vi "Begin.vi"(8 "error in":errorcluster) -> (0 "error out":errorcluster)   [LabVIEW 2019]
doc: "Called before other user functions, this VI is expected to open initial I/O refnums, load in file data, and do all program initialization. Notice that the <B>error out</B> terminal is simply used for data flow. Wiring it to other structures or subVIs ensures that this VI runs first."
uses:
  <vilib>/Rock Robotics/WPI/Camera/WPI_CameraImageSize.ctl
  <vilib>/Rock Robotics/WPI/DriverStation/WPI_DriverStationRobotMode2.ctl
  <vilib>/Rock Robotics/WPI/Joystick/WPI_JoystickDeviceEnum.ctl
  <vilib>/Rock Robotics/SystemInterfaces/DIO/FPGA_DIOChannel.ctl
  <vilib>/Rock Robotics/WPI/Encoder/WPI_EncoderType.ctl
  <vilib>/Rock Robotics/WPI/Solenoid/WPI_SolenoidChannel.ctl
  <vilib>/Rock Robotics/WPI/Solenoid/WPI_SolenoidValue.ctl
  <vilib>/Rock Robotics/WPI/SafetyOutput/WPI_SafetyOutputConfigMenu.ctl
  <vilib>/Rock Robotics/WPI/Camera/WPI_CameraFrameRate.ctl
  <vilib>/Rock Robotics/WPI/Camera/WPI_CameraWhite Balance Values.ctl
  <vilib>/Rock Robotics/WPI/Camera/WPI_CameraExposure Values.ctl
  Robot Global Data.vi
  <vilib>/Rock Robotics/Network Tables/NT Write String Array.vi
  <vilib>/Rock Robotics/WPI/Counter/WPI_CounterDigitalInputToDigitalSource.vi
  <vilib>/Rock Robotics/WPI/Solenoid/WPI_SolenoidOpenDouble.vi
  <vilib>/Rock Robotics/WPI/Solenoid/WPI_SolenoidSetEnum.vi
  <vilib>/Rock Robotics/WPI/RobotDrive/WPI_RobotDriveOpen4MotorWithExistingMotors.vi
  <vilib>/Rock Robotics/WPI/Utilities/WPI_GetSetVariantRefNum.vi
panel:
  in  "Image Size":T1=enum."320x240"
  in  "Image Size 2":T1=enum."320x240"
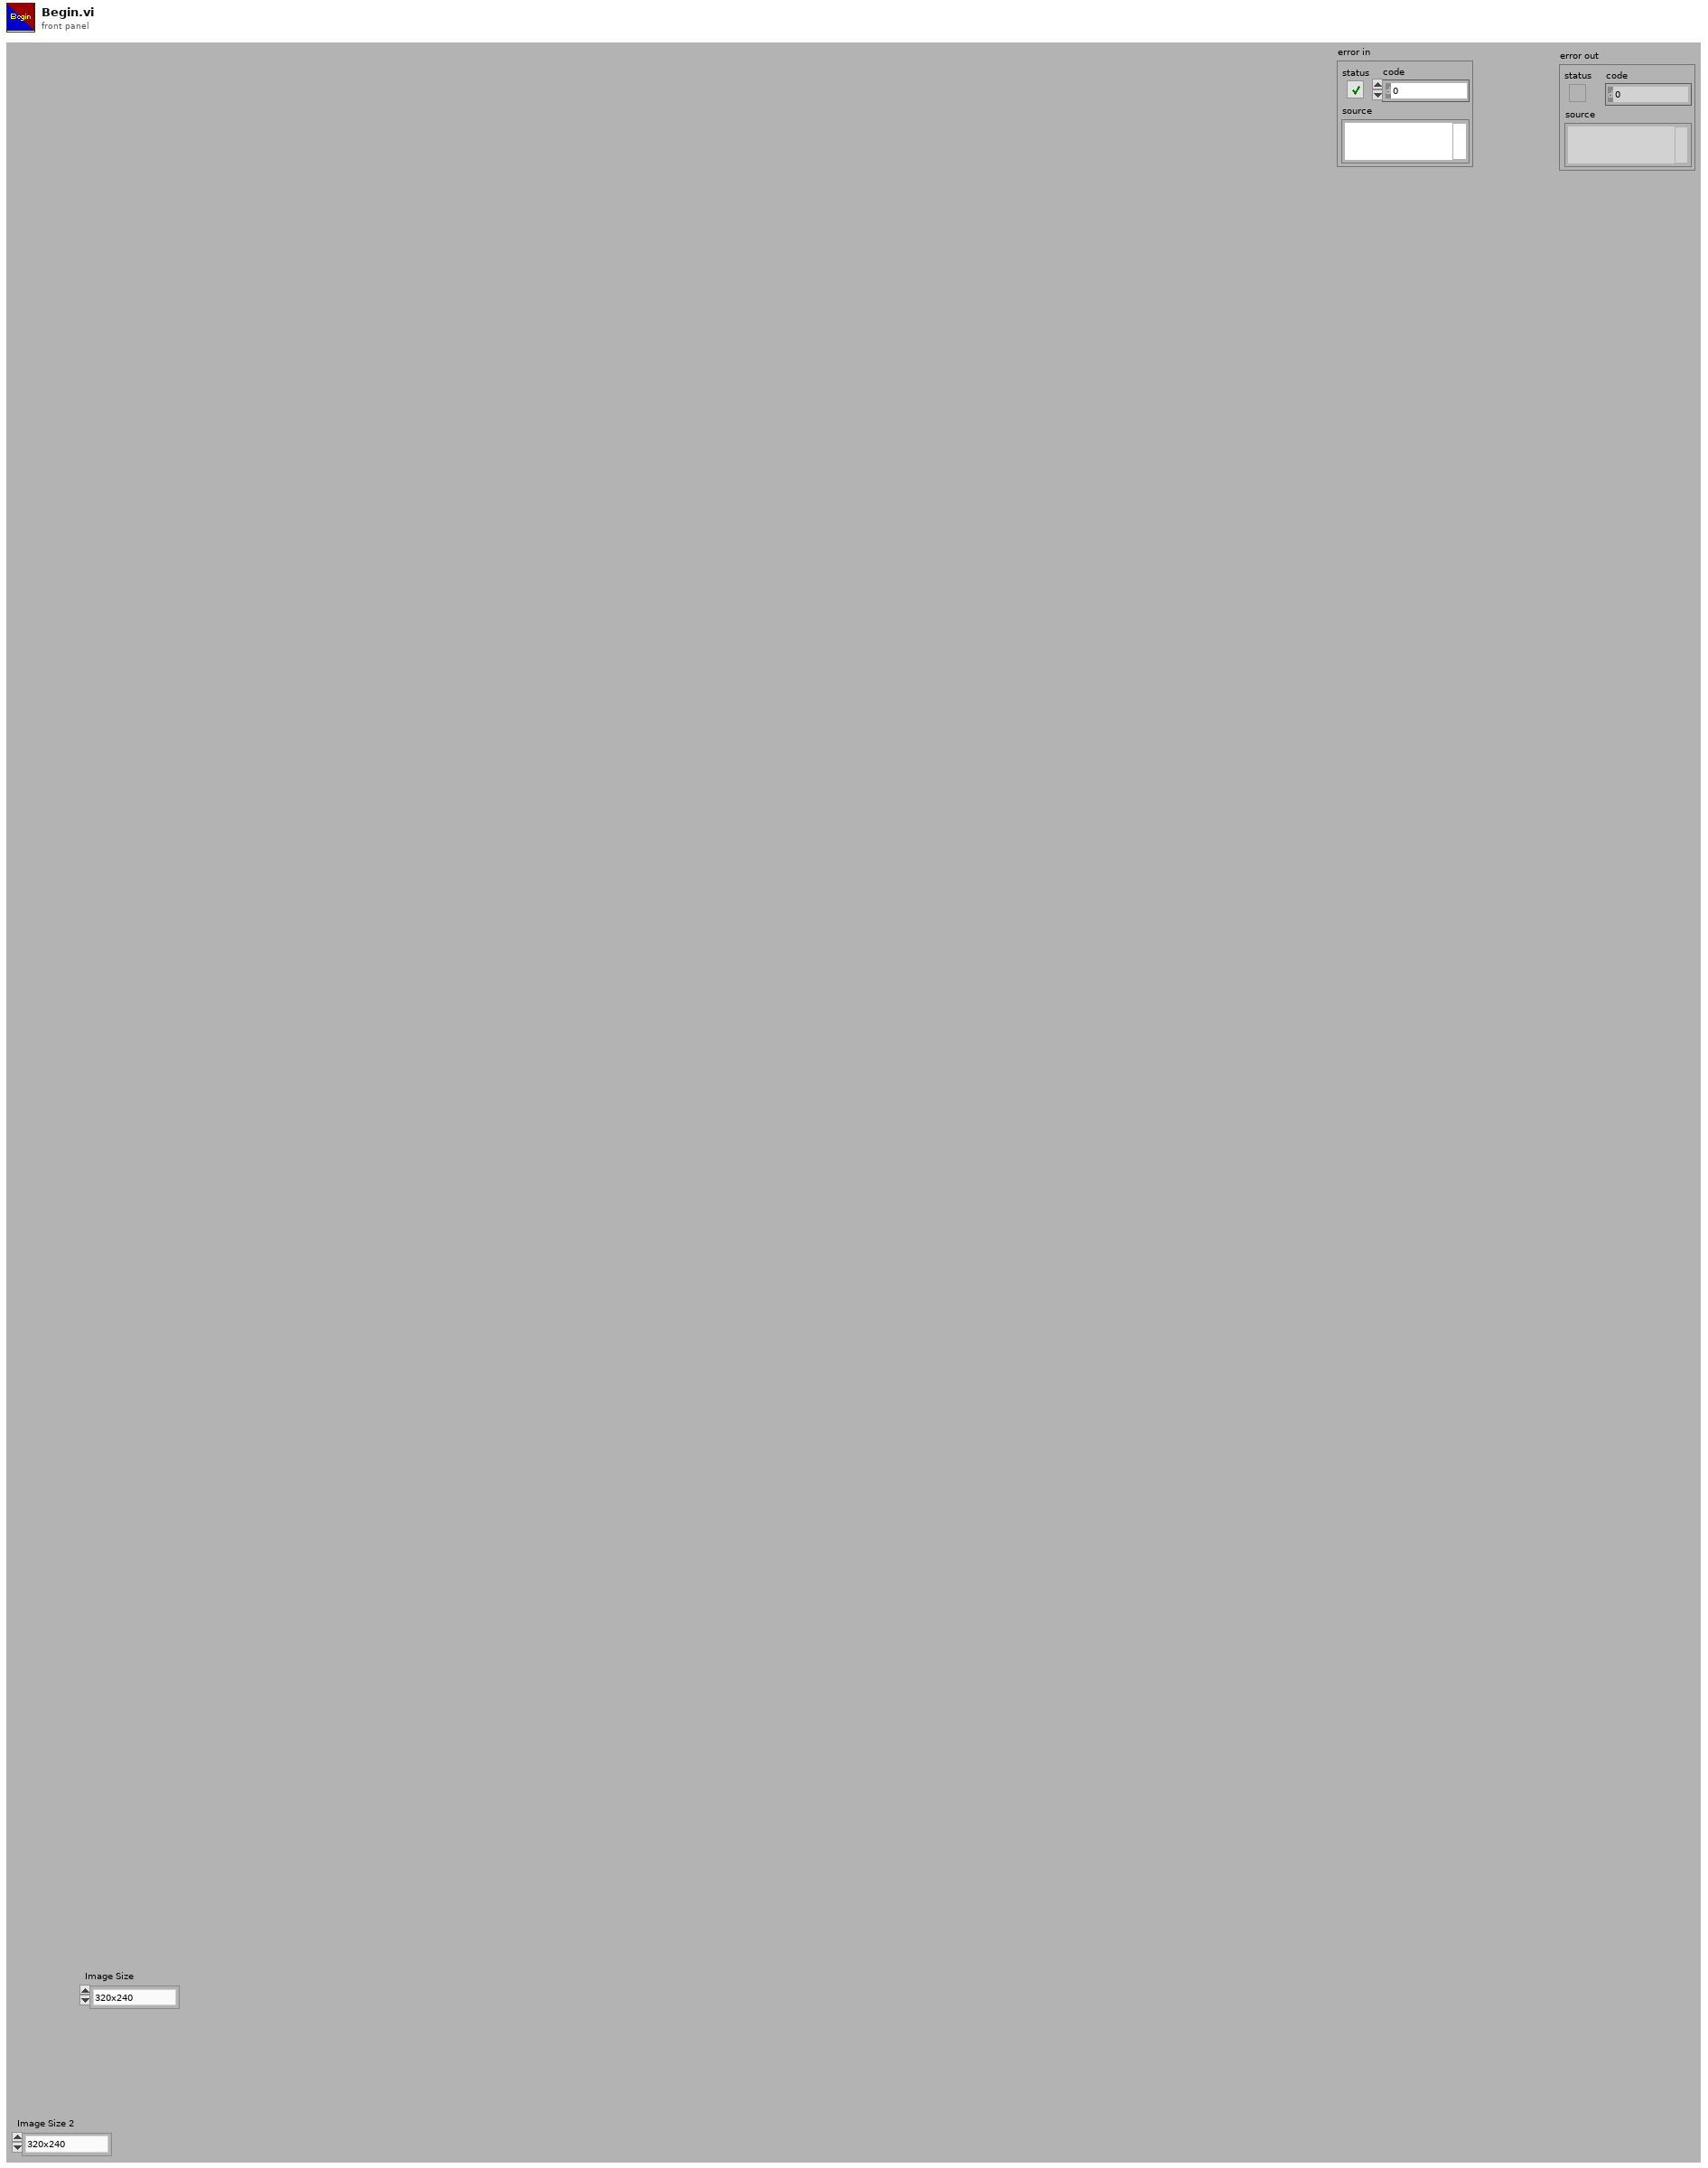
[diagram p1: front panel]
types:
  T1 = typedef "WPI_CameraImageSize.ctl" = enum16{"640x480", "320x240", "160x120", "Custom"}
  T2 = typedef "WPI_CameraFrameRate.ctl" = u32
  T3 = typedef "WPI_CameraExposure Values.ctl" = enum16{"Auto", "Flicker-free 50 Hz", "Flicker-free 60 Hz", "Hold current", "Custom"}
  T4 = typedef "WPI_CameraWhite Balance Values.ctl" = enum16{"Auto", "Fixed indoor", "Fixed outdoor 1", "Fixed outdoor 2", "Fixed fluorescent 1", "Fixed fluorescent 2", "Hold current", "Custom"}
  T5 = typedef "WPI_SolenoidValue.ctl" = enum16{"Off", "On", "Forward", "Reverse"}
  T6 = typedef "WPI_SolenoidChannel.ctl" = enum8{"Solenoid 0", "Solenoid 1", "Solenoid 2", "Solenoid 3", "Solenoid 4", "Solenoid 5", "Solenoid 6", "Solenoid 7", "Invalid"}
  T7 = typedef "WPI_JoystickDeviceEnum.ctl" = enum16{"USB 0", "USB 1", "USB 2", "USB 3", "USB 4", "USB 5"}
  T8 = typedef "WPI_SafetyOutputConfigMenu.ctl" = enum16{"Enable", "Disable"}
  T9 = typedef "WPI_EncoderType.ctl" = enum16{"1x", "2x", "4x"}
  T10 = typedef "FPGA_DIOChannel.ctl" = enum8{"DIO 0", "DIO 1", "DIO 2", "DIO 3", "DIO 4", "DIO 5", "DIO 6", "DIO 7", "DIO 8", "DIO 9", "DIO MXP 0", "DIO MXP 1", "DIO MXP 2", "DIO MXP 3", "DIO MXP 4", "DIO MXP 5", "DIO MXP 6", "DIO MXP 7", "DIO MXP 8", "DIO MXP 9", "DIO MXP 10", "DIO MXP 11", "DIO MXP 12", "DIO MXP 13", "DIO MXP 14", "DIO MXP 15", "SPI Port CS1", "SPI Port CS2", "SPI Port CS3", "SPI Port MISO", "SPI Port MOSI", "Invalid"}
  T11 = typedef "WPI_DriverStationRobotMode2.ctl" = enum16{"Autonomous Disabled", "Autonomous Enabled", "Teleop Disabled", "Teleop Enabled", "Disconnected", "Finish", "Test Disabled", "Test Enabled", "Emergency Stopped"}
  T12 = typedef "WPI_JoystickDevRef.ctl" = cluster{"Device":T7}
  T13 = typedef "WPI_SolenoidDevRef.ctl" = cluster{"DevStatus":errorcluster, "Pneumatics Control Module":u8, "Forward Solenoid Channel":T6, "Reverse Solenoid Channel":T6}
  T14 = typedef "WPI_CameraDevRef.ctl" = cluster{"Camera Address":string, "CameraStatus":errorcluster}
  T15 = typedef "WPI_MotorControlDeviceRef.ctl" = cluster{"DeviceStatus":errorcluster, "Type":T16, "PWM":cluster{"PWM Channel":T17, "DeadBand":T18}, "CAN":cluster{"Device Number":u8, "SetOutput VI Ref":variant, "GetOutput VI Ref":variant, "Enable VI Ref":variant, "Disable VI Ref":variant, "Data":variant}, "Invert":bool, "DIO PWM":cluster{"PWM \"Enable\" Channel":T17, "DIOChannel":T10, "PWM Rate":dbl}}
  T16 = typedef "WPI_MotorControlType.ctl" = enum16{"PWM", "CAN", "DIO PWM"}
  T17 = typedef "FPGA_DIOPWMChannel.ctl" = enum8{"PWM 0", "PWM 1", "PWM 2", "PWM 3", "PWM 4", "PWM 5", "PWM 6", "PWM 7", "PWM 8", "PWM 9", "PWM MXP 0", "PWM MXP 1", "PWM MXP 2", "PWM MXP 3", "PWM MXP 4", "PWM MXP 5", "PWM MXP 6", "PWM MXP 7", "PWM MXP 8", "PWM MXP 9", "Invalid"}
  T18 = typedef "WPI_PWMDeadband.ctl" = cluster{"Name":string, "maxPositivePwm":i32, "minPositivePwm":i32, "centerPwm":i32, "maxNegativePwm":i32, "minNegativePwm":i32, "angularRange":u16}
  T19 = typedef "WPI_CompressorDevRef.ctl" = cluster{"DevStatus":errorcluster, "Pneumatics Control Module":u8}
  T20 = typedef "WPI_DigitalInputDevRef.ctl" = cluster{"DevStatus":errorcluster, "DIO Channel":T10}
  T21 = typedef "WPI_RobotDriveDevRef.ctl" = cluster{"DevStatus":errorcluster, "Motors[]":T15[], "Square Inputs":bool, "Max Output":dbl}
  T22 = typedef "FPGA_CounterEncoderSourceConvertionLVSourceType.ctl" = cluster{"DevStatus":errorcluster, "AnalogTriggerMode?":bool, "DigitalMode":cluster{"DIO Channel":T23}, "AnalogTriggerMode":cluster{"AnalogTriggerIndex":T24, "OutputType":T25}}
  T23 = typedef "FPGA_DIODigitalSourceChannel.ctl" = enum8{"DIO 0", "DIO 1", "DIO 2", "DIO 3", "DIO 4", "DIO 5", "DIO 6", "DIO 7", "DIO 8", "DIO 9", "DIO MXP 0", "DIO MXP 1", "DIO MXP 2", "DIO MXP 3", "DIO MXP 4", "DIO MXP 5", "DIO MXP 6", "DIO MXP 7", "DIO MXP 8", "DIO MXP 9", "DIO MXP 10", "DIO MXP 11", "DIO MXP 12", "DIO MXP 13", "DIO MXP 14", "DIO MXP 15", "SPI Port CS1", "SPI Port CS2", "SPI Port CS3", "SPI Port MISO", "SPI Port MOSI", "Disabled"}
  T24 = typedef "FPGA_AnalogTriggerIndex.ctl" = enum8{"Trig 0", "Trig 1", "Trig 2", "Trig 3", "Trig 4", "Trig 5", "Trig 6", "Trig 7", "Invalid"}
  T25 = typedef "FPGA_AnalogTriggerOutType.ctl" = enum16{"InWindow", "TriggerState", "Rising", "Falling"}
  T26 = typedef "WPI_EncoderDevRef.ctl" = cluster{"DevStatus":errorcluster, "EncoderIndex":T27, "CounterIndex":T28, "DistancePerCount":dbl, "Decoding Type":T9}
  T27 = typedef "FPGA_EncoderIdx.ctl" = enum8{"Enc 0", "Enc 1", "Enc 2", "Enc 3", "Enc 4", "Enc 5", "Enc 6", "Enc 7", "Invalid"}
  T28 = typedef "FPGA_CounterCtrSystemIndex.ctl" = enum8{"Ctr 0", "Ctr 1", "Ctr 2", "Ctr 3", "Ctr 4", "Ctr 5", "Ctr 6", "Ctr 7", "Invalid"}
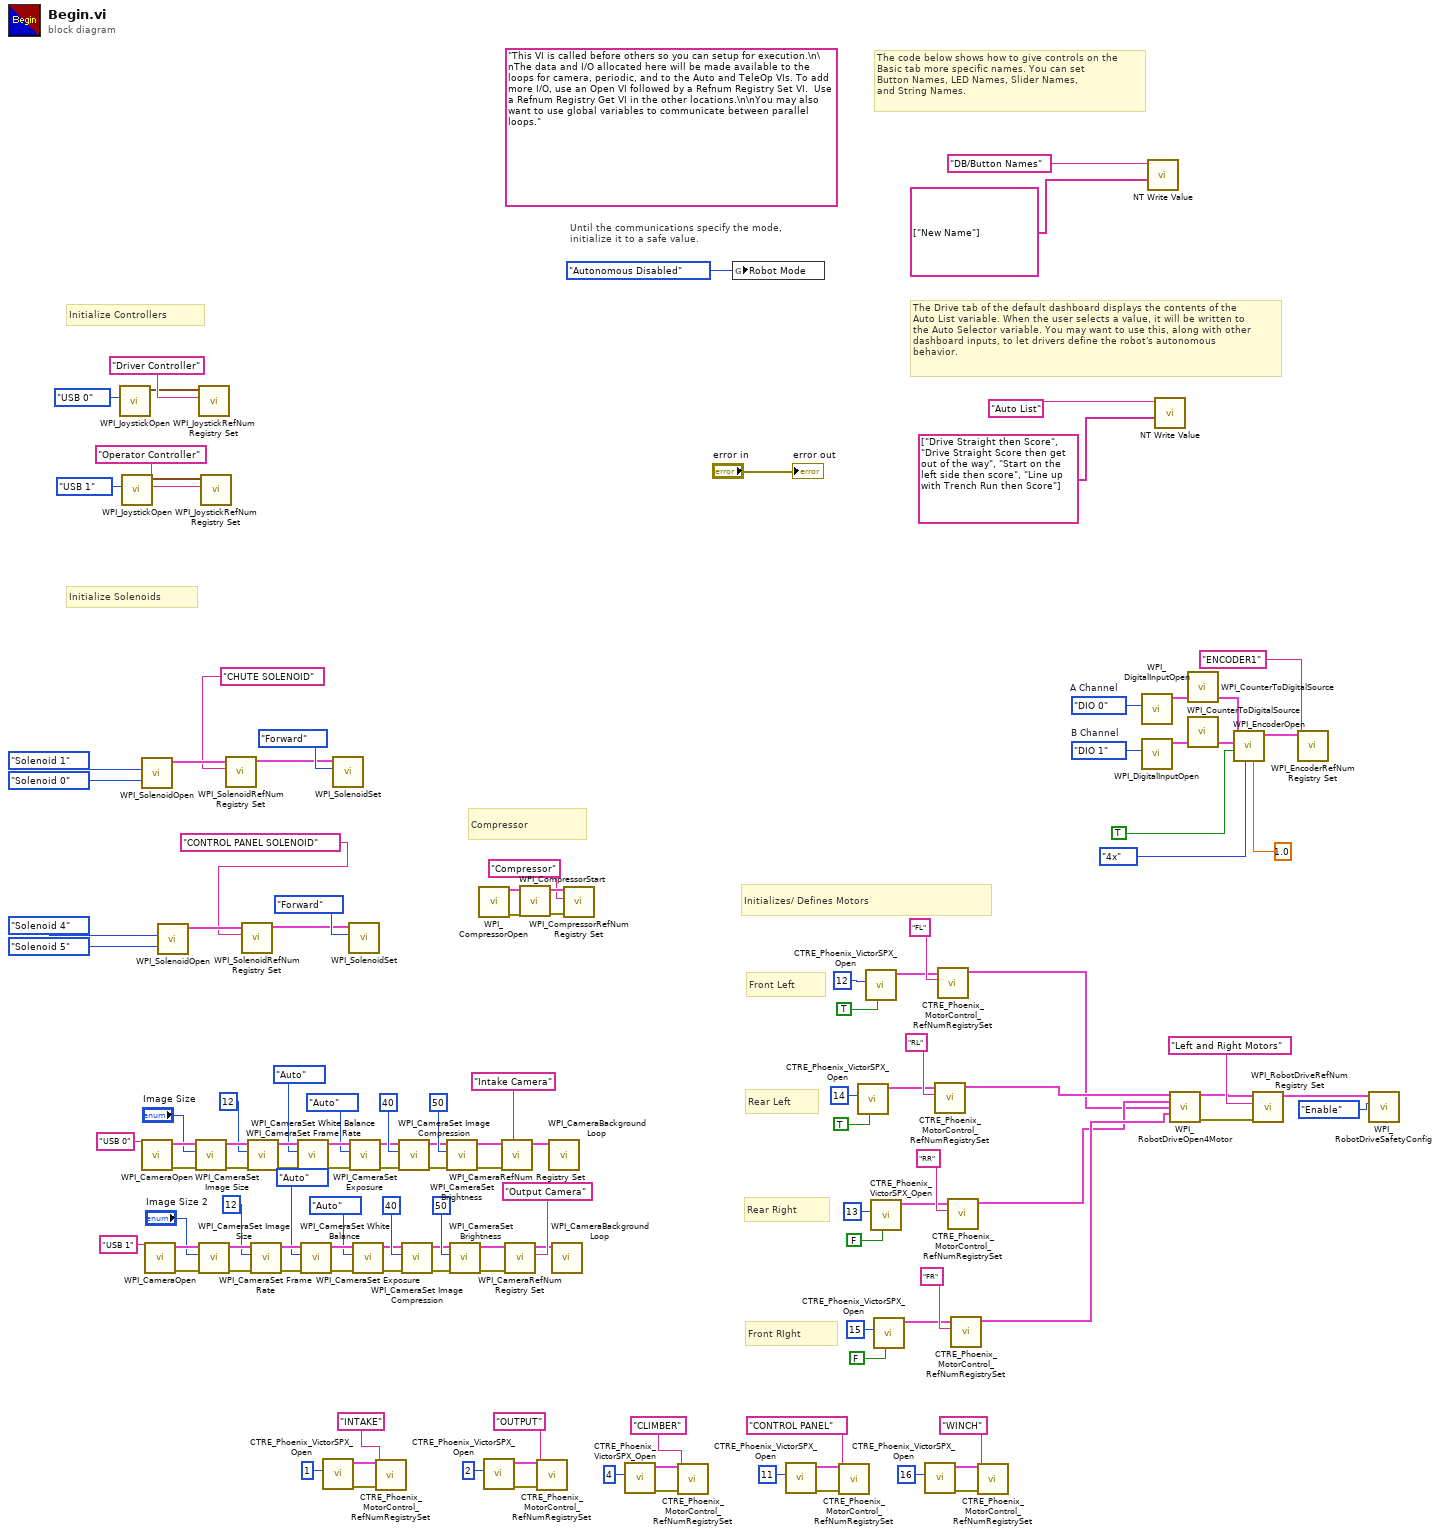
[diagram p0: block diagram]
diagram:
  w122 = FPGA_DIOChannel."DIO 1"  # B Channel
  w121 = FPGA_DIOChannel."DIO 0"  # A Channel
  (unwired) "This VI is called before others so you can setup for execution.\n\nThe data and I/O allocated here will be made available to the loops for camera, periodic, and to the Auto and TeleOp VIs. To add more I/O, use an Open VI followed by a Refnum Registry Set VI.  Use a Refnum Registry Get VI in the other locations.\n\nYou may also want to use global variables to communicate between parallel loops."
  # "Initialize Solenoids"
  # "Front RIght"
  # "Rear Right"
  # "Rear Left"
  # "Front Left"
  # "Initializes/ Defines Motors"
  # "Compressor"
  # "The Drive tab of the default dashboard displays the contents of the\nAuto List variable. When the user selects a value, it will be written to\nthe Auto Selector variable. You may want to use this, along with other\ndashboard inputs, to let drivers define the robot's autonomous\nbehavior."
  # "The code below shows how to give controls on the\nBasic tab more specific names. You can set\nButton Names, LED Names, Slider Names,\nand String Names."
  # "Initialize Controllers"
  # "Until the communications specify the mode,\ninitialize it to a safe value."
  n1 = call <vilib>:"WPI_JoystickOpen.vi"("JoystickDevice"=WPI_JoystickDeviceEnum."USB 0") -> ("JoystickDevRef"=w129:T12)  [unwired: 10 in]
  n2 = call <vilib>:"WPI_JoystickOpen.vi"("JoystickDevice"=WPI_JoystickDeviceEnum."USB 1") -> ("JoystickDevRef"=w66:T12)  [unwired: 10 in]
  n3 = call-poly <vilib>:"WPI_SolenoidOpen.vi"("Reverse Solenoid Channel"=WPI_SolenoidChannel."Solenoid 0", "Forward Solenoid Channel"=WPI_SolenoidChannel."Solenoid 1") -> ("SolenoidDevRef"=w111:T13)  [unwired: 8 in, 1 out]
  n4 = call <vilib>:"WPI_CameraOpen.vi"("Camera Address"="USB 0" ("format string")) -> ("error out"=w37:errorcluster, "CameraDevRef"=w38:T14)  [unwired: 1 in, 8 out]
  n5 = call <vilib>:"WPI_CameraOpen.vi"("Camera Address"="USB 1" ("format string")) -> ("error out"=w14:errorcluster, "CameraDevRef"=w15:T14)  [unwired: 1 in, 8 out]
  n6 = call-poly <vilib>:"WPI_SolenoidOpen.vi"("Reverse Solenoid Channel"=WPI_SolenoidChannel."Solenoid 5", "Forward Solenoid Channel"=WPI_SolenoidChannel."Solenoid 4") -> ("SolenoidDevRef"=w52:T13)  [unwired: 8 in, 1 out]
  n7 = call <vilib>:"WPI_CameraSet Image Size.vi"("error in (no error)"=w37, "Image Size"="Image Size", "CameraDevRef"=w38) -> ("error out"=w36:errorcluster, "CameraDevRef Out"=w39:T14)  [unwired: 1 in, 6 out]
  n8 = call <vilib>:"WPI_JoystickRefNum Registry Set.vi"("refnum name"="Driver Controller", "JoystickDevRef"=w129) -> ()  [unwired: 8 in, 2 out]
  n9 = call <vilib>:"WPI_CameraSet Image Size.vi"("error in (no error)"=w14, "Image Size"="Image Size 2", "CameraDevRef"=w15) -> ("error out"=w13:errorcluster, "CameraDevRef Out"=w16:T14)  [unwired: 1 in, 6 out]
  n10 = call <vilib>:"WPI_JoystickRefNum Registry Set.vi"("refnum name"="Operator Controller", "JoystickDevRef"=w66) -> ()  [unwired: 8 in, 2 out]
  n11 = call <vilib>:"WPI_SolenoidRefNum Registry Set.vi"("refnum name"="CHUTE SOLENOID", "SolenoidDevRef"=w111) -> ("SolenoidDevRef"=w101:T13)  [unwired: 8 in, 1 out]
  n12 = call <vilib>:"WPI_SolenoidRefNum Registry Set.vi"("refnum name"="CONTROL PANEL SOLENOID", "SolenoidDevRef"=w52) -> ("SolenoidDevRef"=w48:T13)  [unwired: 8 in, 1 out]
  n13 = call <vilib>:"WPI_CameraSet Frame Rate.vi"("error in (no error)"=w36, "Frame Rate (fps)"=T2 12, "CameraDevRef"=w39) -> ("error out"=w35:errorcluster, "CameraDevRef Out"=w41:T14)  [unwired: 7 out]
  n14 = call <vilib>:"WPI_CameraSet Frame Rate.vi"("error in (no error)"=w13, "Frame Rate (fps)"=T2 12, "CameraDevRef"=w16) -> ("error out"=w12:errorcluster, "CameraDevRef Out"=w18:T14)  [unwired: 7 out]
  n15 = call <vilib>:"WPI_CameraSet White Balance.vi"("error in (no error)"=w35, "White Balance"=WPI_CameraWhite_Balance_Values."Auto", "CameraDevRef"=w41) -> ("error out"=w34:errorcluster, "CameraDevRef Out"=w40:T14)  [unwired: 1 in, 6 out]
  n16 = call <vilib>:"WPI_CameraSet White Balance.vi"("error in (no error)"=w12, "White Balance"=WPI_CameraWhite_Balance_Values."Auto", "CameraDevRef"=w18) -> ("error out"=w11:errorcluster, "CameraDevRef Out"=w17:T14)  [unwired: 1 in, 6 out]
  n17 = call <vilib>:"CTRE_Phoenix_VictorSPX_Open.vi"("Device Number"=u8 1) -> ("error out"=w74:errorcluster, "CAN Talon SRX Ref"=w73:T15)  [unwired: 9 in]
  n18 = call-poly <vilib>:"WPI_SolenoidSet.vi"("Value"=WPI_SolenoidValue."Forward", "SolenoidDevRef"=w101) -> ()  [unwired: 8 in, 2 out]
  n19 = call-poly <vilib>:"WPI_SolenoidSet.vi"("Value"=WPI_SolenoidValue."Forward", "SolenoidDevRef"=w48) -> ()  [unwired: 8 in, 2 out]
  n20 = call <vilib>:"WPI_CameraSet Exposure.vi"("error in (no error)"=w34, "Exposure"=WPI_CameraExposure_Values."Auto", "CameraDevRef"=w40) -> ("error out"=w33:errorcluster, "CameraDevRef Out"=w43:T14)  [unwired: 1 in, 6 out]
  n21 = call <vilib>:"WPI_CameraSet Exposure.vi"("error in (no error)"=w11, "Exposure"=WPI_CameraExposure_Values."Auto", "CameraDevRef"=w17) -> ("error out"=w10:errorcluster, "CameraDevRef Out"=w20:T14)  [unwired: 1 in, 6 out]
  n22 = call <vilib>:"CTRE_Phoenix_MotorControl_RefNumRegistrySet.vi"("error in (no error)"=w74, "refnum name"="INTAKE", "PhoenixMotorControlDevRef"=w73) -> ()  [unwired: 7 in, 2 out]
  n23 = call <vilib>:"WPI_CameraSet Image Compression.vi"("error in (no error)"=w33, "Compression"=40, "CameraDevRef"=w43) -> ("error out"=w32:errorcluster, "CameraDevRef Out"=w42:T14)  [unwired: 7 out]
  n24 = call <vilib>:"WPI_CameraSet Image Compression.vi"("error in (no error)"=w10, "Compression"=40, "CameraDevRef"=w20) -> ("error out"=w9:errorcluster, "CameraDevRef Out"=w19:T14)  [unwired: 7 out]
  n25 = call <vilib>:"WPI_CameraSet Brightness.vi"("error in (no error)"=w32, "Brightness"=50, "CameraDevRef"=w42) -> ("error out"=w30:errorcluster, "CameraDevRef Out"=w31:T14)  [unwired: 1 in, 6 out]
  n26 = call <vilib>:"WPI_CameraSet Brightness.vi"("error in (no error)"=w9, "Brightness"=50, "CameraDevRef"=w19) -> ("error out"=w7:errorcluster, "CameraDevRef Out"=w8:T14)  [unwired: 1 in, 6 out]
  n27 = call <vilib>:"WPI_CompressorOpen.vi"() -> ("CompressorDevRef"=w106:T19, "error out"=w107:errorcluster)  [unwired: 14 in]
  n28 = call <vilib>:"CTRE_Phoenix_VictorSPX_Open.vi"("Device Number"=u8 2) -> ("error out"=w70:errorcluster, "CAN Talon SRX Ref"=w69:T15)  [unwired: 9 in]
  n29 = call <vilib>:"WPI_CameraRefNum Registry Set.vi"("error in (no error)"=w30, "refnum name"="Intake Camera", "CameraDevRef"=w31) -> ("CameraDevRef"=w26:T14)  [unwired: 1 in, 7 out]
  n30 = call <vilib>:"WPI_CameraRefNum Registry Set.vi"("error in (no error)"=w7, "refnum name"="Output Camera", "CameraDevRef"=w8) -> ("CameraDevRef"=w3:T14)  [unwired: 1 in, 7 out]
  n31 = call <vilib>:"WPI_CompressorStart.vi"("error in (no error)"=w107, "CompressorDevRef"=w106) -> ("error out"=w105:errorcluster, "CompressorDevRef"=w104:T19)  [unwired: 8 in]
  n32 = call <vilib>:"CTRE_Phoenix_MotorControl_RefNumRegistrySet.vi"("error in (no error)"=w70, "refnum name"="OUTPUT", "PhoenixMotorControlDevRef"=w69) -> ()  [unwired: 7 in, 2 out]
  n33 = call <vilib>:"WPI_CameraBackground Loop.vi"("CameraDevRef"=w26) -> ()  [unwired: 11 in]
  n34 = call <vilib>:"WPI_CameraBackground Loop.vi"("CameraDevRef"=w3) -> ()  [unwired: 11 in]
  n35 = call <vilib>:"WPI_CompressorRefNum Registry Set.vi"("error in (no error)"=w105, "refnum name"="Compressor", "CompressorDevRef"=w104) -> ()  [unwired: 7 in, 2 out]
  n36 = call <vilib>:"CTRE_Phoenix_VictorSPX_Open.vi"("Device Number"=u8 4) -> ("error out"=w63:errorcluster, "CAN Talon SRX Ref"=w62:T15)  [unwired: 9 in]
  n37 = call <vilib>:"CTRE_Phoenix_MotorControl_RefNumRegistrySet.vi"("error in (no error)"=w63, "refnum name"="CLIMBER", "PhoenixMotorControlDevRef"=w62) -> ()  [unwired: 7 in, 2 out]
  n38 = global write "Robot Global Data.vi" "Robot Mode"(WPI_DriverStationRobotMode2."Autonomous Disabled" ("Robot Mode")) -> ()
  n39 = call <vilib>:"CTRE_Phoenix_VictorSPX_Open.vi"("Device Number"=u8 11) -> ("error out"=w59:errorcluster, "CAN Talon SRX Ref"=w58:T15)  [unwired: 9 in]
  n40 = call <vilib>:"CTRE_Phoenix_MotorControl_RefNumRegistrySet.vi"("error in (no error)"=w59, "refnum name"="CONTROL PANEL", "PhoenixMotorControlDevRef"=w58) -> ()  [unwired: 7 in, 2 out]
  n41 = call <vilib>:"CTRE_Phoenix_VictorSPX_Open.vi"("Invert"=TRUE, "Device Number"=u8 14) -> ("CAN Talon SRX Ref"=w76:T15)  [unwired: 8 in, 1 out]
  n42 = call <vilib>:"CTRE_Phoenix_VictorSPX_Open.vi"("Invert"=TRUE, "Device Number"=u8 12) -> ("CAN Talon SRX Ref"=w83:T15)  [unwired: 8 in, 1 out]
  n43 = call <vilib>:"CTRE_Phoenix_VictorSPX_Open.vi"("Invert"=FALSE, "Device Number"=u8 13) -> ("CAN Talon SRX Ref"=w86:T15)  [unwired: 8 in, 1 out]
  n44 = call <vilib>:"CTRE_Phoenix_VictorSPX_Open.vi"("Invert"=FALSE, "Device Number"=u8 15) -> ("CAN Talon SRX Ref"=w89:T15)  [unwired: 8 in, 1 out]
  n45 = call <vilib>:"CTRE_Phoenix_VictorSPX_Open.vi"("Device Number"=u8 16) -> ("error out"=w55:errorcluster, "CAN Talon SRX Ref"=w54:T15)  [unwired: 9 in]
  n46 = call <vilib>:"CTRE_Phoenix_MotorControl_RefNumRegistrySet.vi"("refnum name"="RL", "PhoenixMotorControlDevRef"=w76) -> ("PhoenixMotorControlDevRef"=w93:T15)  [unwired: 8 in, 1 out]
  n47 = call <vilib>:"CTRE_Phoenix_MotorControl_RefNumRegistrySet.vi"("refnum name"="FL", "PhoenixMotorControlDevRef"=w83) -> ("PhoenixMotorControlDevRef"=w92:T15)  [unwired: 8 in, 1 out]
  n48 = call <vilib>:"CTRE_Phoenix_MotorControl_RefNumRegistrySet.vi"("refnum name"="RR", "PhoenixMotorControlDevRef"=w86) -> ("PhoenixMotorControlDevRef"=w94:T15)  [unwired: 8 in, 1 out]
  n49 = call <vilib>:"CTRE_Phoenix_MotorControl_RefNumRegistrySet.vi"("refnum name"="FR", "PhoenixMotorControlDevRef"=w89) -> ("PhoenixMotorControlDevRef"=w95:T15)  [unwired: 8 in, 1 out]
  n50 = call <vilib>:"CTRE_Phoenix_MotorControl_RefNumRegistrySet.vi"("error in (no error)"=w55, "refnum name"="WINCH", "PhoenixMotorControlDevRef"=w54) -> ()  [unwired: 7 in, 2 out]
  n51 = call <vilib>:"WPI_DigitalInputOpen.vi"("DIO Channel"=w121) -> ("DigitalInputDevRef"=w118:T20)  [unwired: 1 in, 9 out]
  n52 = call <vilib>:"WPI_DigitalInputOpen.vi"("DIO Channel"=w122) -> ("DigitalInputDevRef"=w119:T20)  [unwired: 1 in, 9 out]
  n53 = call-poly <vilib>:"NT Write Value.vi"("String Array"=string[] ["New Name"], "Name"="DB/Button Names") -> ()  [unwired: 9 in, 1 out]
  n54 = call-poly <vilib>:"NT Write Value.vi"("String Array"=string[] ["Drive Straight then Score", "Drive Straight Score then get out of the way", "Start on the left side then score", "Line up with Trench Run then Score"], "Name"="Auto List") -> ()  [unwired: 9 in, 1 out]
  n55 = call-poly <vilib>:"WPI_RobotDriveOpen4Motor.vi"("Rear Left Motor Dev Ref"=w93, "Rear Right Motor Dev Ref"=w94, "Front Left Motor Dev Ref"=w92, "Front Right Motor Dev Ref"=w95) -> ("RobotDriveDevRef"=w79:T21, "error out"=w81:errorcluster)  [unwired: 10 in]
  n56 = call-poly <vilib>:"WPI_CounterToDigitalSource.vi"("DigitalInputDevRef"=w118) -> ("Digital Source"=w117:T22)  [unwired: 6 out]
  n57 = call-poly <vilib>:"WPI_CounterToDigitalSource.vi"("DigitalInputDevRef"=w119) -> ("Digital Source"=w120:T22)  [unwired: 6 out]
  n58 = call <vilib>:"WPI_EncoderOpen.vi"("DistancePerCount"=1.0, "Decoding Type"=WPI_EncoderType."4x", "Invert Direction (False)"=TRUE, "BSource"=w120, "ASource"=w117) -> ("EncoderDevRef"=w113:T26)  [unwired: 3 in, 3 out]
  n59 = call <vilib>:"WPI_RobotDriveRefNum Registry Set.vi"("error in (no error)"=w81, "refnum name"="Left and Right Motors", "RobotDriveDevRef"=w79) -> ("RobotDriveDevRef"=w82:T21)  [unwired: 1 in, 7 out]
  n60 = call <vilib>:"WPI_EncoderRefNum Registry Set.vi"("refnum name"="ENCODER1", "EncoderDevRef"=w113) -> ()  [unwired: 8 in, 2 out]
  n61 = call <vilib>:"WPI_RobotDriveSafetyConfig.vi"("mode"=WPI_SafetyOutputConfigMenu."Enable", "RobotDriveDevRef"=w82) -> ()  [unwired: 8 in, 2 out]
  "error out" <- "error in"
